vi "TestRUSH.vi"() -> ()   [LabVIEW 2012]
panel:
  out "HarvOutRollerB":dbl
  out "HarvOutRollerF":dbl
  out "HarvShootEnable":bool
  out "HarvOutElev":dbl
  in  "HarvClustIn":T1 {"HarvPOTElev" scale=0.0..5.0; "HarvManualElev" scale=-1.0..1.0; "HarvRollerBDesSpd" scale=-1.0..1.0; "HarvRollerFDesSpd" scale=-1.0..1.0}
  in  "LowerLimit":bool
  in  "UpperLimit":bool
  in  "HarvSetElev":i32
  in  "HarvPOTElev":dbl(knob) scale=0.0..5.0
  in  "HarvManualElev":dbl(slide) scale=-1.0..1.0
  in  "HarvRollerBDesSpd":dbl(slide) scale=-1.0..1.0
  in  "HarvRollerFDesSpd":dbl(slide) scale=-1.0..1.0
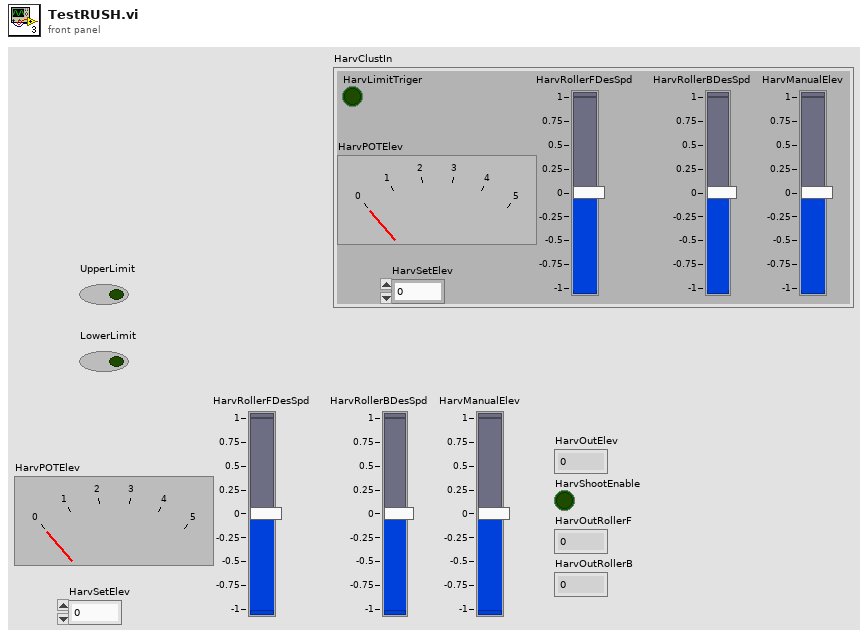
[diagram p1: front panel]
types:
  T1 = cluster{"HarvLimitTriger":bool, "HarvRollerFDesSpd":dbl, "HarvRollerBDesSpd":dbl, "HarvManualElev":dbl, "HarvPOTElev":dbl, "HarvSetElev":i32}
  T2 = cluster{"HarvOutElev":dbl, "HarvShootEnable":bool, "HarvOutRollerF":dbl, "HarvOutRollerB":dbl}
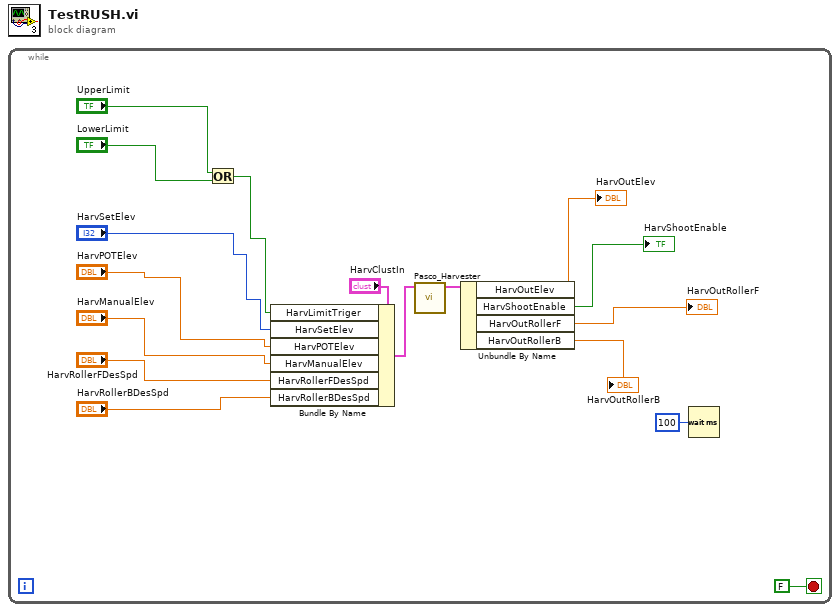
[diagram p0: block diagram]
diagram:
  n1 = while {
    stop <- FALSE stop-if-true
    n2 = Or(x="UpperLimit", y="LowerLimit") -> (x .or. y?=w10:bool)
    n3 = Bundle By Name(cluster="HarvClustIn", "HarvLimitTriger"=w10, "HarvSetElev"="HarvSetElev", "HarvPOTElev"="HarvPOTElev", "HarvManualElev"="HarvManualElev", "HarvRollerFDesSpd"="HarvRollerFDesSpd", "HarvRollerBDesSpd"="HarvRollerBDesSpd") -> (w11:T1)
    n4 = call "Pasco_Harvester.vi"("HarvClustIn"=w11) -> ("HarvClustOut"=w15:T2)  [unwired: 10 in]
    n5 = Unbundle By Name(w15) -> ("HarvOutElev"=→"HarvOutElev":dbl, "HarvShootEnable"=→"HarvShootEnable":bool, "HarvOutRollerF"=→"HarvOutRollerF":dbl, "HarvOutRollerB"=→"HarvOutRollerB":dbl)
    n6 = Wait (ms)(milliseconds to wait=u32 100) -> ()  [unwired: 1 out]
  }
